vi "readAO.vi"(8 "error in (no error)":errorcluster, 11 "Instrument.Lockin in":refnum<class "Instrument.Lockin.lvclass">) -> (0 "error out":errorcluster, 2 "AO Waveforrm":waveform(dbl)[](array[waveform]), 3 "Instrument.Lockin out":refnum<class "Instrument.Lockin.lvclass">)   [LabVIEW 2016, in "Instrument.Lockin.lvclass"]
doc: "API to get the AO waveforms.\n\nIf address=\"\", this API reads from localhost\nIf address is remote lockin, you need to add this computer to allowed whitelist on the lockin computer you are trying to access."
uses:
  Instrument.Lockin.lvclass
  Typedefs/Instrument.Lockin.Commands--Enum.ctl
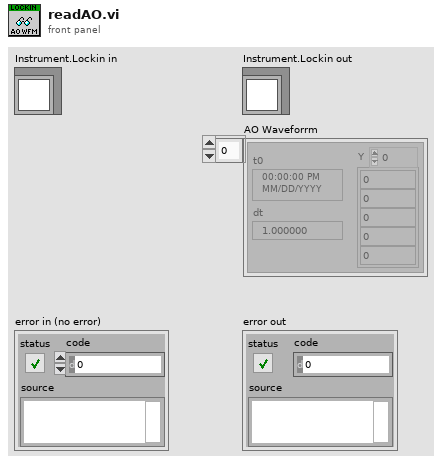
[diagram p1: front panel]
types:
  T1 = typedef "Instrument.Lockin.lvclass/Instrument.Lockin.Commands--Enum.ctl" = enum16{"configAO", "configAO_Amplitude", "configAO_DC", "configAO_Frequency", "configAO_Phase", "configAO_Function", "configAO_I+", "configREF", "configREF_Frequency", "configREF_Phase", "configREF_Filter", "configIVmode", "Reset", "configSampling", "Trigger", "getAO", "getAI", "getResults", "getTrigger", "getIVmode", "getSampling", "getAOconfig", "getREFconfig", "getREF_Filter", "configGain", "getGain", "configAutoSampling", "getAutoSampling"}
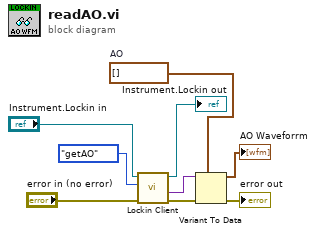
[diagram p0: block diagram]
diagram:
  w4 = waveform(dbl)[] []  # AO
  n1 = call "Lockin Client.vi"("error in (no error)"="error in (no error)", "Command"=Instrument.Lockin.Commands--Enum."getAO", "Instrument.Lockin in"="Instrument.Lockin in") -> ("error out"=w8:errorcluster, "Data out"=w9:variant, "Instrument.Lockin out"=→"Instrument.Lockin out":refnum<class "Instrument.Lockin.lvclass">)  [unwired: 6 in]
  n2 = Variant To Data(error in=w8, type=w4, Variant=w9) -> (data=→"AO Waveforrm":waveform(dbl)[], error out=→"error out":errorcluster)
